vi "Command (read & write) - IF.vi"(7 "timeout ms (100)":i32=100, 8 "error in (no error)":errorcluster, 9 "Format":string, 10 "IP":string, 11 "connection ID in":refnum<k16>) -> (0 "error out":errorcluster, 3 "connection ID out":refnum<k16>)   [LabVIEW 2016, in "SMD-7615.lvlib" / "eSCL.lvlib"]
doc: "IF - Immediate Format\nSets the data format, hexadecimal or decimal, for data returned using all “I” commands (except IH, IL, IO and IS).Data can be requested from the drive in two formats: hexadecimal or decimal. By default data is returned in hexadecimal because of its speed and efficiency. Conversion to ascii in the decimal format is slower and causes a slight delay that varies in length. Hexadecimal minimizes the overhead required to convert the internal binary data to ascii form. This speeds up the process of sending out the requested data thus giving the most recent value. Typically, applications written on more powerful host computers can easily convert a hexadecimal value into a decimal value.\nAll “I” commands can be used at any time and at the fastest rate possible limited only by the given baud rate (see BR and PB commands). Immediate commands are executed as they are received, regardless of what is in the drive’s command buffer. Regardless of format (hex or dec) there will be a slight delay in processing the response to an “I” command. “Real time” usage of the data must be carefully analyzed."
uses:
  eSCL.lvlib
  String Command and Param.ctl
panel:
  out "Format":string
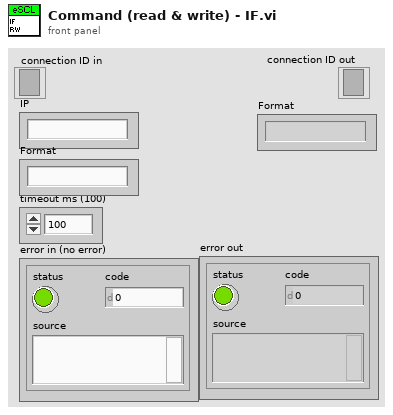
[diagram p1: front panel]
types:
  T1 = typedef "SMD-7615.lvlib/eSCL.lvlib/String Command and Param.ctl" = cluster{"Command":string, "String Parameler":string, "String Parameler Default":string}
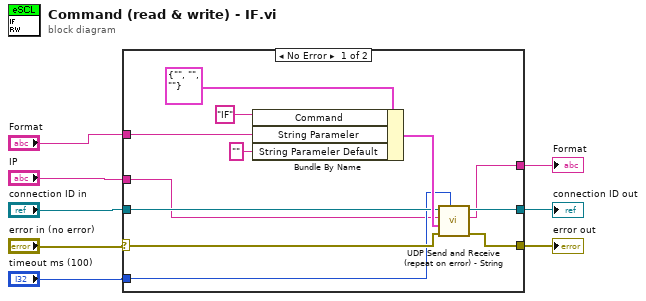
[diagram p0: block diagram]
diagram:
  n1 = case shown="No Error" "error in (no error)" {
    selector: "error in (no error)" -> [w16 w21]
    tunnel: "connection ID in" -> [w14 w22]
    tunnel: [w18 w22] -> w2
    tunnel: [w17 w21] -> w1
    tunnel: "IP" -> [w12 _]
    tunnel: "timeout ms (100)" -> [w13 _]
    tunnel: "Format" -> [w11 _]
    tunnel: [w9 _] -> w8
    frame No Error {
      n2 = Bundle By Name(cluster=T1 {"Command"="", "String Parameler"="", "String Parameler Default"=""} ("String Command & Param"), "Command"="IF", "String Parameler"=w11, "String Parameler Default"="") -> (w15:T1)
      n3 = call "UDP Send and Receive (repeat on error) - String.vi"("timeout ms (100)"=w13, "error in (no error)"=w16, "String Command & Param"=w15, "IP"=w12, "connection ID in"=w14) -> ("error out"=w17:errorcluster, "String Param out"=w9:string, "connection ID out"=w18:refnum<k16>)  [unwired: 4 in]
    }
    frame Error {
    }
  }
  "connection ID out" <- w2
  "error out" <- w1
  "Format" <- w8
